vi "CLD 7 Time Stamp to Initialization String Solution.vi"(8 "Fehler (Eingang)":T1) -> (0 "Fehler (Ausgang)":T1, 3 "Code-String (Ausgang)":string)   [LabVIEW 2014]
doc: "CLD 7: Die zusätzlichen Anzeigeelemente dienen der Fehlersuche. \n\nBei Lösungen, in denen nicht der Zeitstempel im US-Format verwendet wird, verläuft das Parsing etwas anders. Dieses Lösungs-VI wurde für einen Zeitstempel im US-Format entwickelt. Ein Schalter stellt zwei Strings zur Verfügung, die von einem Zeitstempel im US-Format ausgegeben werden."
panel:
  in  "Schalter (Internationales Format)":bool
  out "Jahr":string
  out "Tag":string
  out "Monat":string
  out "Wochentag":string
  out "AM/PM":string
  out "Sekunden":string
  out "Minuten":string
  out "Stunde":string
  out "Datum":string
  out "Zeit":string
  # "Anzeigeelemente zur Fehlersuche unten"
  # "Für US-Zeitstempel auf FALSE setzen\nFür internationale Zeitstempel auf TRUE setzen"
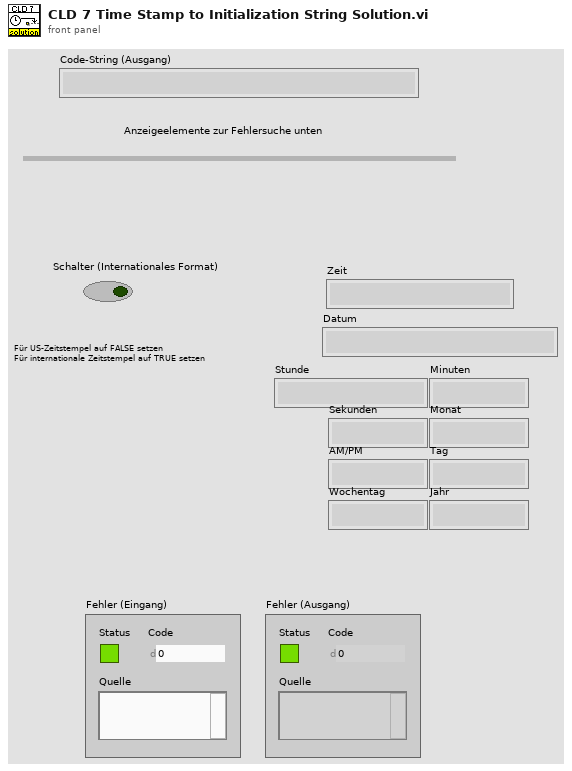
[diagram p1: front panel]
types:
  T1 = cluster{"Status":bool, "Code":i32, "Quelle":string}
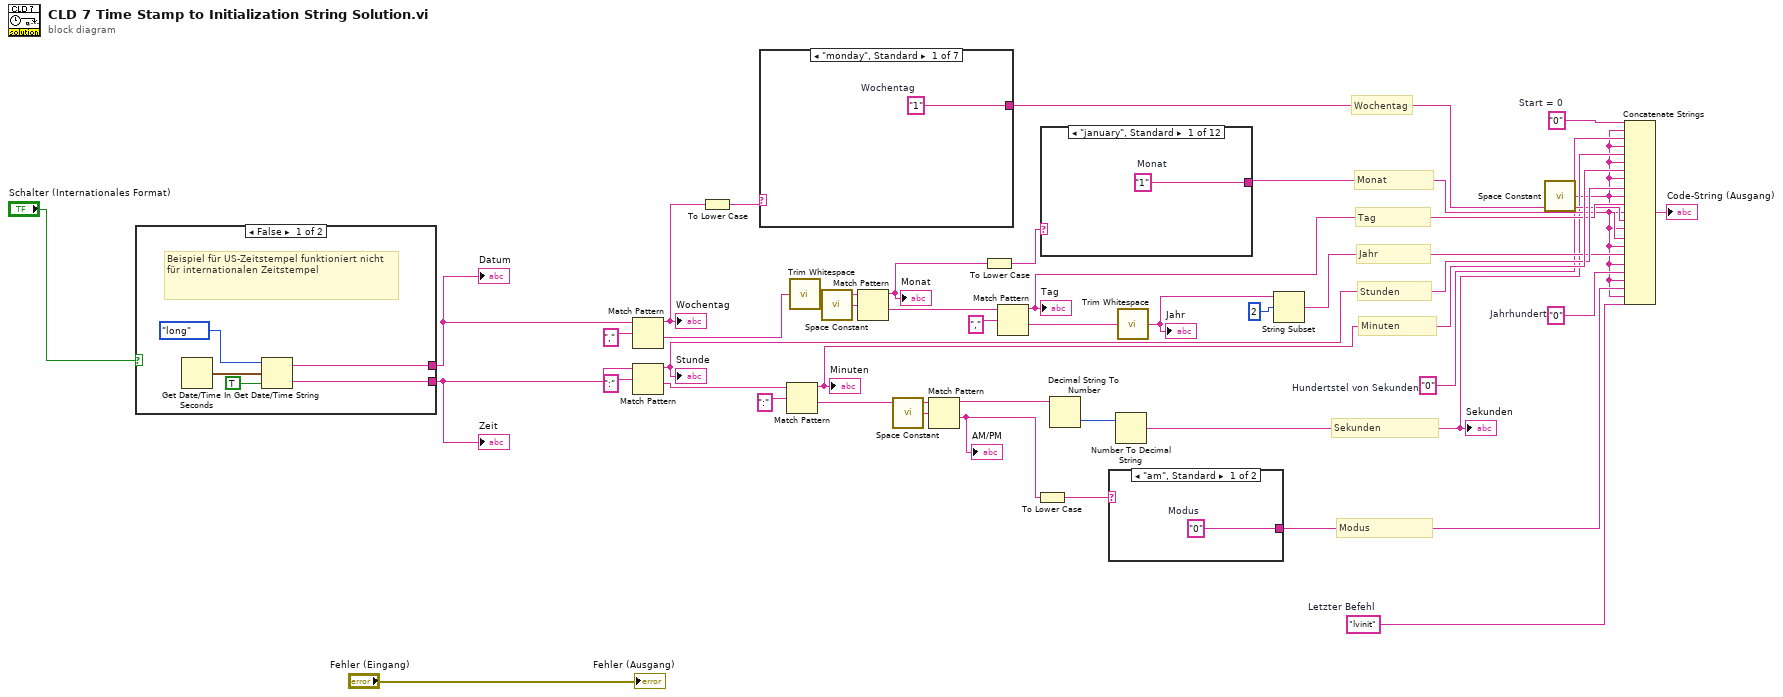
[diagram p0: block diagram]
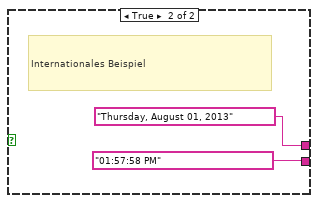
[diagram p2: hidden frame]
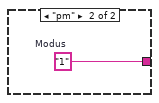
[diagram p3: hidden frame]
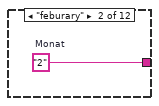
[diagram p4: hidden frame]
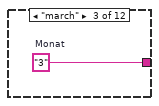
[diagram p5: hidden frame]
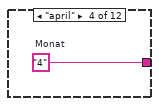
[diagram p6: hidden frame]
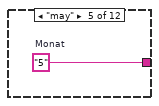
[diagram p7: hidden frame]
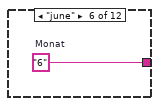
[diagram p8: hidden frame]
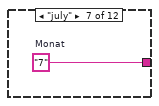
[diagram p9: hidden frame]
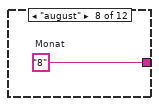
[diagram p10: hidden frame]
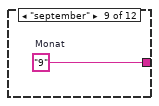
[diagram p11: hidden frame]
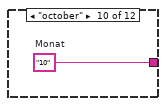
[diagram p12: hidden frame]
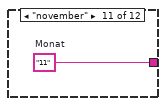
[diagram p13: hidden frame]
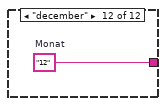
[diagram p14: hidden frame]
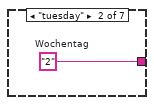
[diagram p15: hidden frame]
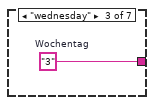
[diagram p16: hidden frame]
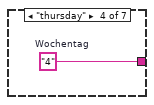
[diagram p17: hidden frame]
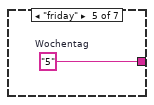
[diagram p18: hidden frame]
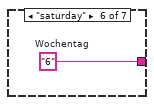
[diagram p19: hidden frame]
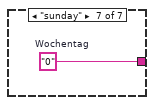
[diagram p20: hidden frame]
diagram:
  w7 = "0"  # Start = 0
  w14 = "0"  # Jahrhundert
  w3 = "0"  # Hundertstel von Sekunden
  w8 = "lvinit"  # Letzter Befehl
  # "Minuten"
  # "Stunden"
  # "Tag"
  # "Wochentag"
  # "Monat"
  # "Jahr"
  # "Modus"
  # "Sekunden"
  n1 = case shown="False" "Schalter (Internationales Format)" {
    tunnel: [w42 "01:57:58 PM"] -> w35
    tunnel: [w41 "Thursday, August 01, 2013"] -> w27
    frame False {
      # "Beispiel für US-Zeitstempel funktioniert nicht für internationalen Zeitstempel"
      n2 = Get Date/Time In Seconds() -> (seconds since 1Jan1904=w45:timestamp)
      n3 = Get Date/Time String(date format (0)=enum16{"short", "long", "abbreviated"}."long" ("Datumsformat (0)"), seconds (now)=w45, want seconds? (F)=TRUE ("Angabe von Sekunden? (F)")) -> (date string=w41:string, time string=w42:string)
    }
    frame True {
      # "Internationales Beispiel"
    }
  }
  "Zeit" <- w35
  "Datum" <- w27
  n4 = Match Pattern(string=w27, regular expression="," ("Regulärer Ausdruck")) -> (before substring=w23:string, after substring=w33:string)  [unwired: 1 in, 2 out]
  "Wochentag" <- w23
  n5 = Match Pattern(string=w35, regular expression=":" ("Regulärer Ausdruck")) -> (before substring=w25:string, after substring=w38:string)  [unwired: 1 in, 2 out]
  "Stunde" <- w25
  n6 = To Lower Case(string=w23) -> (all lower case string=w22:string)
  n7 = case shown="\"monday\", Standard" w22 {
    tunnel: [w48 w49 w50 w51 w52 w53 w54] -> w21
    frame "monday", Default {
      w48 = "1"  # Wochentag
    }
    frame "tuesday" {
      w49 = "2"  # Wochentag
    }
    frame "wednesday" {
      w50 = "3"  # Wochentag
    }
    frame "thursday" {
      w51 = "4"  # Wochentag
    }
    frame "friday" {
      w52 = "5"  # Wochentag
    }
    frame "saturday" {
      w53 = "6"  # Wochentag
    }
    frame "sunday" {
      w54 = "0"  # Wochentag
    }
  }
  n8 = Match Pattern(string=w38, regular expression=":" ("Regulärer Ausdruck")) -> (before substring=w26:string, after substring=w37:string)  [unwired: 1 in, 2 out]
  "Minuten" <- w26
  n9 = call <vilib>:"Trim Whitespace.vi"("string"=w33) -> ("trimmed string"=w32:string)  [unwired: 1 in]
  n10 = call <vilib>:"Space Constant.vi"() -> ("String"=w31:string)
  n11 = Match Pattern(string=w32, regular expression=w31) -> (before substring=w20:string, after substring=w29:string)  [unwired: 1 in, 2 out]
  "Monat" <- w20
  n12 = call <vilib>:"Space Constant.vi"() -> ("String"=w36:string)
  n13 = Match Pattern(string=w37, regular expression=w36) -> (before substring=w5:string, after substring=w13:string)  [unwired: 1 in, 2 out]
  "AM/PM" <- w13
  n14 = To Lower Case(string=w20) -> (all lower case string=w19:string)
  n15 = Match Pattern(string=w29, regular expression="," ("Regulärer Ausdruck")) -> (before substring=w24:string, after substring=w28:string)  [unwired: 1 in, 2 out]
  "Tag" <- w24
  n16 = To Lower Case(string=w13) -> (all lower case string=w12:string)
  n17 = case shown="\"january\", Standard" w19 {
    tunnel: [w55 w56 w57 w58 w59 w60 w61 w62 w63 w64 w65 w66] -> w18
    frame "january", Default {
      w55 = "1"  # Monat
    }
    frame "feburary" {
      w56 = "2"  # Monat
    }
    frame "march" {
      w57 = "3"  # Monat
    }
    frame "april" {
      w58 = "4"  # Monat
    }
    frame "may" {
      w59 = "5"  # Monat
    }
    frame "june" {
      w60 = "6"  # Monat
    }
    frame "july" {
      w61 = "7"  # Monat
    }
    frame "august" {
      w62 = "8"  # Monat
    }
    frame "september" {
      w63 = "9"  # Monat
    }
    frame "october" {
      w64 = "10"  # Monat
    }
    frame "november" {
      w65 = "11"  # Monat
    }
    frame "december" {
      w66 = "12"  # Monat
    }
  }
  n18 = Decimal String To Number(string=w5) -> (number=w6:i32)  [unwired: 2 in, 1 out]
  n19 = case shown="\"am\", Standard" w12 {
    tunnel: [w67 w68] -> w11
    frame "am", Default {
      w67 = "0"  # Modus
    }
    frame "pm" {
      w68 = "1"  # Modus
    }
  }
  n20 = Number To Decimal String(number=w6) -> (decimal integer string=w4:string)  [unwired: 1 in]
  "Sekunden" <- w4
  n21 = call <vilib>:"Trim Whitespace.vi"("string"=w28) -> ("trimmed string"=w17:string)  [unwired: 1 in]
  "Jahr" <- w17
  n22 = String Subset(string=w17, offset (0)=2 ("Offset (0)")) -> (substring=w15:string)  [unwired: 1 in]
  n23 = call <vilib>:"Space Constant.vi"() -> ("String"=w2:string)
  n24 = Concatenate Strings(w7, w2, w3, w2, w4, w2, w26, w2, w25, w2, w24, w2, w21, w2, w18, w2, w15, w2, w14, w2, w11, w2, w8) -> (→"Code-String (Ausgang)":string)
  "Fehler (Ausgang)" <- "Fehler (Eingang)"
